vi "Handle Message.vi"(8 "error in (no error)":errorcluster, 9 "Message Completion Handler":refnum<class "Message Completion Handler.lvclass">, 10 "Message":string, 11 "CSV Export in":refnum<class "CSV Export.lvclass">) -> (0 "error out":errorcluster, 1 "Synchronously Complete Message?":bool=TRUE, 2 "Message Response":string, 3 "CSV Export out":refnum<class "CSV Export.lvclass">)   [LabVIEW 2022 SP3, in "CSV Export.lvlib" / "CSV Export.lvclass"]
uses:
  CSV Export.lvclass
  CSV Export.lvclass/CSV Export.ctl
  Global.vi
  <vilib>/FlexLogger/SDK/PluginSDK.lvlibp/PEFClasses/SDK/System Interface/System Interface.lvclass
  <vilib>/FlexLogger/SDK/PluginSDK.lvlibp/PEFClasses/SDK/Message Completion Handler/Message Completion Handler.lvclass
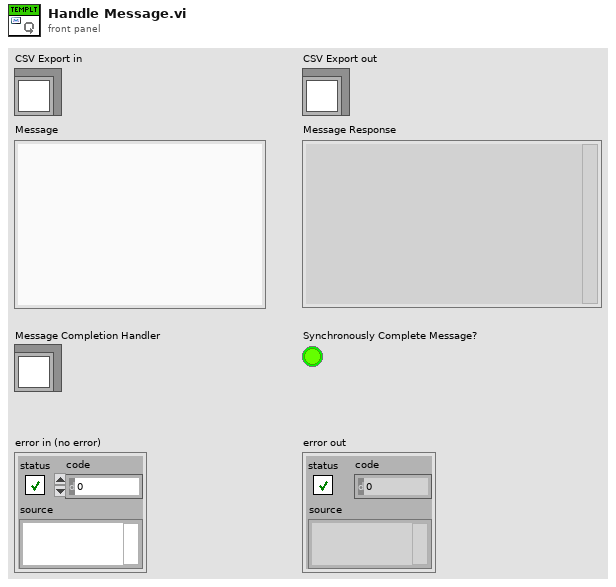
[diagram p1: front panel]
types:
  T1 = typedef "CSV Export.lvlib/CSV Export.lvclass/CSV Export Settings.ctl" = cluster{"Log Stats":bool, "Time Format":string, "Resampled":bool, "Resampled Rate":dbl, "Digits of Precision":u32, "Relative Time":bool}
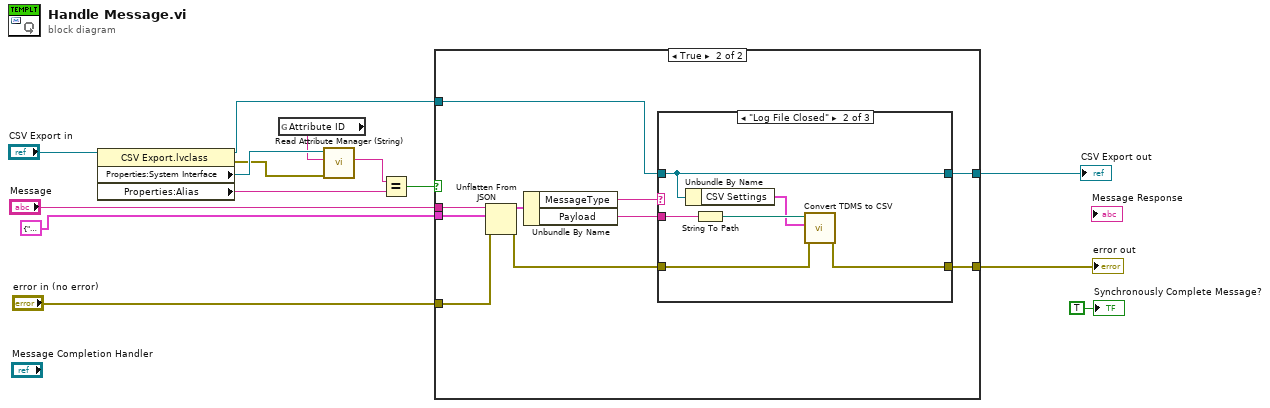
[diagram p0: block diagram]
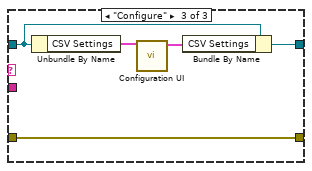
[diagram p4: hidden frame]
diagram:
  n1 = property class="CSV Export.lvclass"(reference="CSV Export in") -> (reference out=w5:refnum<class "CSV Export.lvclass">, error out=w10:errorcluster, "Properties:System Interface"=w11:refnum<class "System Interface.lvclass">, "Properties:Alias"=w6:string)  [unwired: 1 in]
  n2 = global read "Global.vi" "Attribute ID"() -> (w9:string)
  n3 = call-dynamic "Read Attribute Manager (String).vi"("error in (no error)"=w10, "Attribute ID"=w9, "System Interface in"=w11) -> ("Attrib Val"=w7:string)  [unwired: 5 in, 3 out]
  n4 = Equal?(x=w7, y=w6) -> (x = y?=w3:bool)
  n5 = case shown="True" w3 {
    tunnel: cluster{"Payload":string, "MessageType":string} {"Payload"="", "MessageType"=""} -> [_ w26]
    tunnel: "Message" -> [_ w24]
    tunnel: "error in (no error)" -> [w16 w21]
    tunnel: [w16 w19] -> w2
    tunnel: w5 -> [w15 w18]
    tunnel: [w15 w17] -> w1
    frame False {
      # "Let Process.vi report error about this not being the only instance."
    }
    frame True {
      n6 = Unflatten From JSON(JSON string=w24, type and defaults=w26, error in (no error)=w21) -> (value=w25:cluster{"Payload":string, "MessageType":string}, error out=w20:errorcluster)  [unwired: 4 in]
      n7 = Unbundle By Name(w25) -> ("MessageType"=w23:string, "Payload"=w22:string)
      n8 = case shown="\"Log File Closed\"" w23 {
        tunnel: w22 -> [_ w34 _]
        tunnel: w18 -> [w27 w29 w37]
        tunnel: w20 -> [w28 w31 w35]
        tunnel: [w28 w30 w35] -> w19
        tunnel: [w27 w29 w36] -> w17
        frame Default {
        }
        frame "Log File Closed" {
          n9 = Unbundle By Name(w29) -> ("CSV Settings"=w32:T1)
          n10 = String To Path(string=w34) -> (path=w33:path)
          n11 = call "Convert TDMS to CSV.vi"("error in (no error)"=w31, "CSV Settings"=w32, "TDMS File"=w33) -> ("error out"=w30:errorcluster)  [unwired: 8 in]
        }
        frame "Configure" {
          n12 = Unbundle By Name(w37) -> ("CSV Settings"=w39:T1)
          n13 = call "Configuration UI.vi"("CSV Settings In"=w39) -> ("CSV Settings Out"=w38:T1)  [unwired: 10 in]
          n14 = Bundle By Name(cluster=w37, "CSV Settings"=w38) -> (w36:refnum<class "CSV Export.lvclass">)
        }
      }
    }
  }
  "error out" <- w2
  "CSV Export out" <- w1
  "Synchronously Complete Message?" <- TRUE ("Synchronously Complete Message?")
